vi "Simulated VeriStand Engine.Interface.Allocate.Control Pointers.vi"(8 "error in (no error)":errorcluster, 11 "Simulated VeriStand Engine Interface in":refnum<class "Simulated VeriStand Engine.Interface.lvclass">) -> (0 "error out":errorcluster, 3 "Simulated VeriStand Engine Interface out":refnum<class "Simulated VeriStand Engine.Interface.lvclass">)   [LabVIEW 2016, in "Simulated VeriStand Engine.Interface.lvclass"]
uses:
  Simulated VeriStand Engine.Interface.lvclass
  Typedefs/Simulated VeriStand Engine.Interface.Pointers.Control.ctl
  Source/Submodules/Memory/Source/Classes/Internal/Memory.Pointer.Internal.lvclass
  Simulated VeriStand Engine.Interface.lvclass/Simulated VeriStand Engine.Interface.ctl
  Source/Submodules/Memory/Source/Classes/Internal/Memory.Pointer.Internal.Allocate.vi
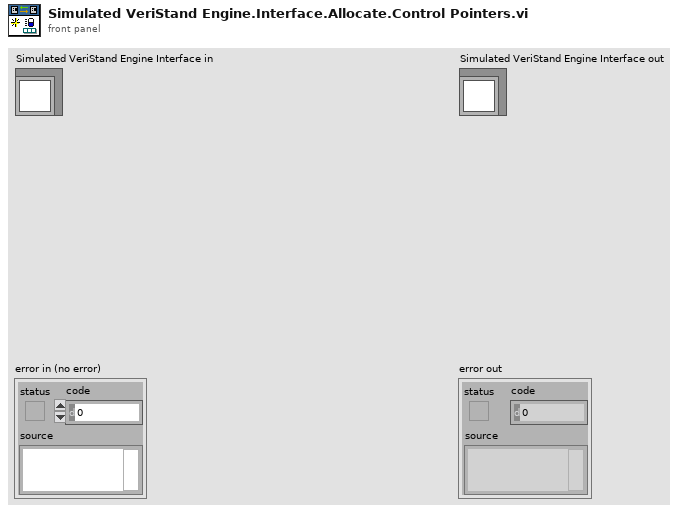
[diagram p1: front panel]
types:
  T1 = typedef "Simulated VeriStand Engine.Interface.lvclass/Simulated VeriStand Engine.Interface.Pointers.Control.ctl" = cluster{"Stop":refnum<class "Memory.Pointer.Internal.lvclass">, "Target Period (µs)":refnum<class "Memory.Pointer.Internal.lvclass">}
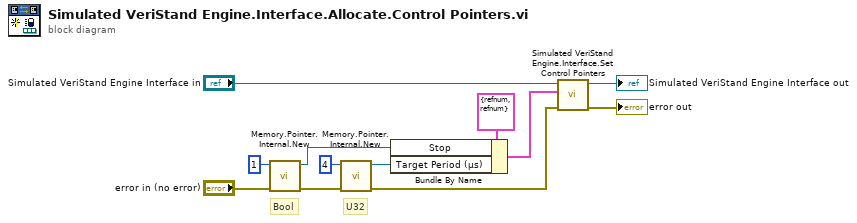
[diagram p0: block diagram]
diagram:
  # "U32"
  # "Bool"
  n1 = call "Memory.Pointer.Internal.New.vi"("error in (no error)"="error in (no error)", "size"=u64 1) -> ("error out"=w6:errorcluster, "pointer"=w9:refnum<class "Memory.Pointer.Internal.lvclass">)  [unwired: 8 in]
  n2 = call "Memory.Pointer.Internal.New.vi"("error in (no error)"=w6, "size"=u64 4) -> ("error out"=w2:errorcluster, "pointer"=w10:refnum<class "Memory.Pointer.Internal.lvclass">)  [unwired: 8 in]
  n3 = Bundle By Name(cluster=T1 {"Stop"=refnum, "Target Period (µs)"=refnum} ("Control Pointers"), "Stop"=w9, "Target Period (µs)"=w10) -> (w11:T1)
  n4 = call "Simulated VeriStand Engine.Interface.Set Control Pointers.vi"("error in (no error)"=w2, "Control Pointers"=w11, "Simulated VeriStand Engine Interface in"="Simulated VeriStand Engine Interface in") -> ("error out"=→"error out":errorcluster, "Simulated VeriStand Engine Interface out"=→"Simulated VeriStand Engine Interface out":refnum<class "Simulated VeriStand Engine.Interface.lvclass">)  [unwired: 7 in]
